vi "test.vi"() -> ()   [LabVIEW 2013]
uses:
  <vilib>/vision/NI_Vision_Development_Module.lvlib
panel:
  out "Image 3":T1(plugin-control)
  out "x < y?":bool
  out "Waveform Chart":dbl(graph)
  out "Image 2":T1(plugin-control)
  in  "AVI File Path":path=path "F:/Camera/15-04-01_18-21-50/eyemovie.avi.avi"
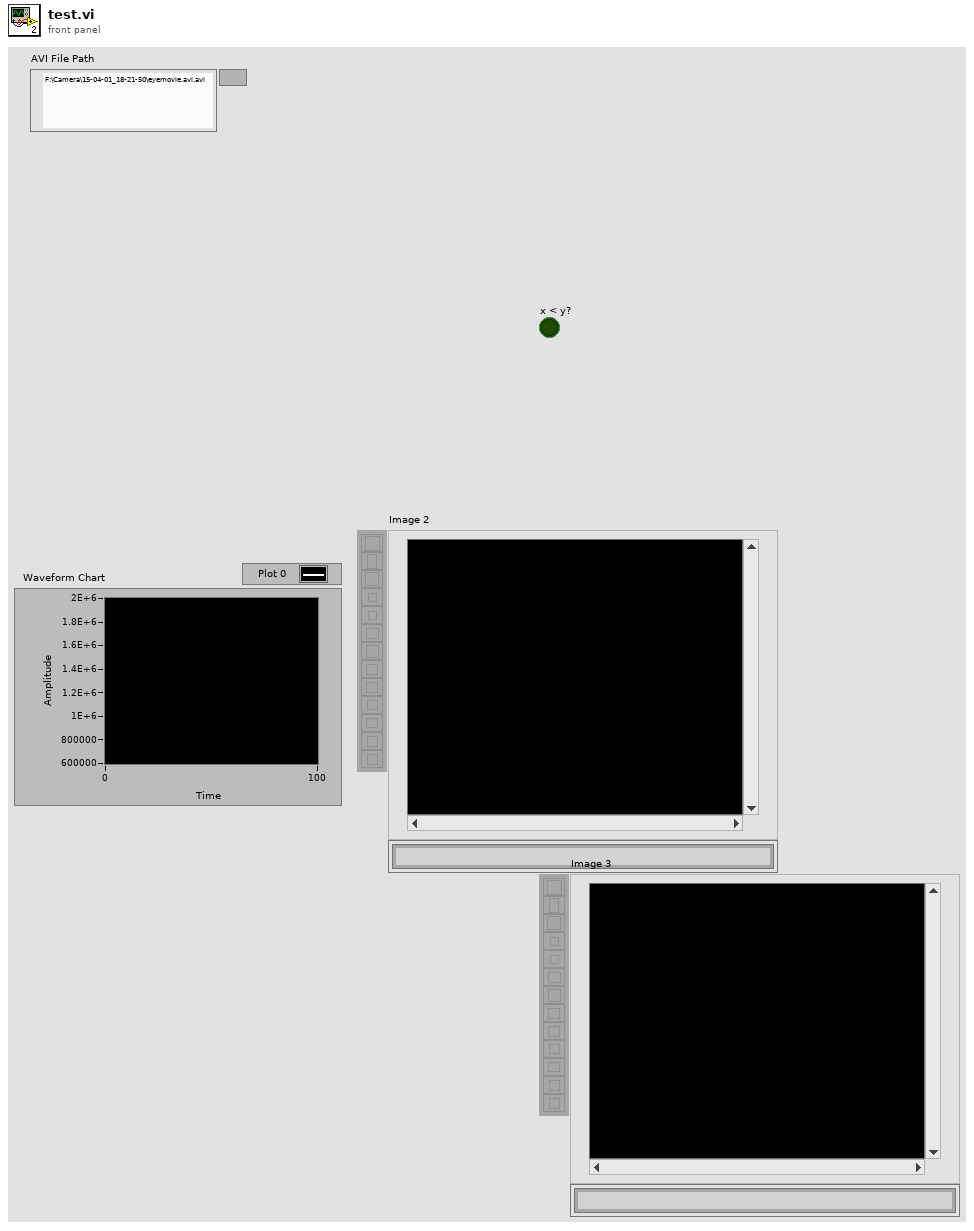
[diagram p1: front panel]
types:
  T1 = typedef "IMAQ Image.ctl" = refnum<image>
  T2 = typedef "IMAQ AVI2 Refnum.ctl" = refnum<k20>
  T3 = cluster{"Global Rectangle":i32[], "Contours":cluster{"Contour Type":u32, "ROI Type":u32, "Points":i32[]}[]}
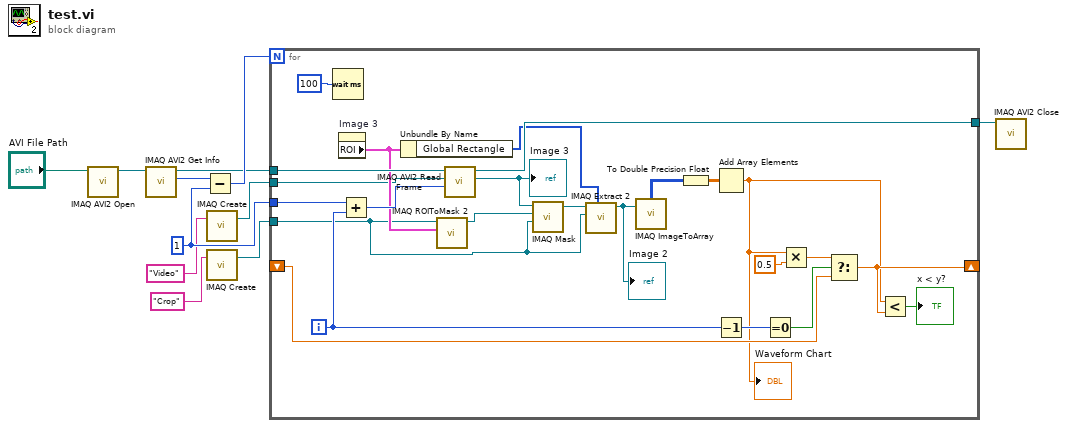
[diagram p0: block diagram]
diagram:
  w6 = 1
  n1 = call "IMAQ AVI2 Open"("AVI File Path"="AVI File Path") -> ("AVI Refnum"=w9:T2)  [unwired: 9 in, 1 out]
  n2 = call "IMAQ AVI2 Get Info"("AVI Refnum"=w9) -> ("Number of Frames"=w8:u32, "AVI Refnum (duplicate)"=w2:T2)  [unwired: 6 in, 3 out]
  n3 = Subtract(x=w8, y=w6) -> (x-y=w7:u32)
  n4 = call "IMAQ Create"("Image Name"="Video") -> ("New Image"=w1:T1)  [unwired: 4 in, 1 out]
  n5 = call "IMAQ Create"("Image Name"="Crop") -> ("New Image"=w3:T1)  [unwired: 4 in, 1 out]
  n6 = for {
    N: w7 -> [_]
    tunnel: [w35] -> w10
    tunnel: w2 -> [w34]
    tunnel: w6 -> [w33]
    tunnel: w3 -> [w12]
    shift-right: [w20] -> _
    shift-left: _ -> [w23]
    tunnel: w1 -> [w14]
    i -> [w22]
    n7 = Wait (ms)(milliseconds to wait=u32 100) -> ()  [unwired: 1 out]
    n8 = property on="Image 3" class="ImageControl"() -> ("ROI"=w16:T3)  [unwired: 2 in, 2 out]
    n9 = Add(x=w33, y=w22) -> (x+y=w32:i32)
    n10 = Unbundle By Name(w16) -> ("Global Rectangle"=w31:i32[])
    n11 = call "IMAQ ROIToMask 2"("ROI Descriptor"=w16, "Image"=w12) -> ("Image Out"=w13:T1)  [unwired: 7 in, 2 out]
    n12 = call "IMAQ AVI2 Read Frame"("Frame Number"=w32, "Image"=w14, "AVI Refnum"=w34) -> ("Image Out"=w15:T1, "AVI Refnum (duplicate)"=w35:T2)  [unwired: 6 in, 1 out]
    "Image 3" <- w15
    n13 = call "IMAQ Mask"("Image Dst"=w12, "Image Mask"=w13, "Image Src"=w15) -> ("Image Dst Out"=w30:T1)  [unwired: 2 in, 1 out]
    n14 = call "IMAQ Extract 2"("Optional Rectangle"=w31, "Image Dst"=w12, "Image Src"=w30) -> ("Image Dst Out"=w29:T1)  [unwired: 7 in, 1 out]
    "Image 2" <- w29
    n15 = call "IMAQ ImageToArray"("Image"=w29) -> ("Image Pixels (U8)"=w26:u8[][])  [unwired: 3 in, 4 out]
    n16 = To Double Precision Float(number=w26) -> (double precision float=w27:dbl[][])
    n17 = Add Array Elements(numeric array=w27) -> (sum=w18:dbl)
    "Waveform Chart" <- w18
    n18 = Decrement(x=w22) -> (x-1=w21:i32)
    n19 = Equal To 0?(x=w21) -> (x = 0?=w24:bool)
    n20 = Multiply(x=w18, y=0.5) -> (x*y=w17:dbl)
    n21 = Select(t=w17, s=w24, f=w23) -> (s? t:f=w20:dbl)
    n22 = Less?(x=w18, y=w20) -> (x < y?=→"x < y?":bool)
  }
  n23 = call "IMAQ AVI2 Close"("AVI Refnum"=w10) -> ()  [unwired: 10 in, 1 out]
